vi "get folders.vi"(8 "error in":errorcluster, 11 "web service in":refnum<vi>) -> (0 "error out":errorcluster, 1 "web methods":refnum<vi>, 2 "startup":refnum<vi>, 3 "Web service project item out":refnum<vi>)   [LabVIEW 2013]
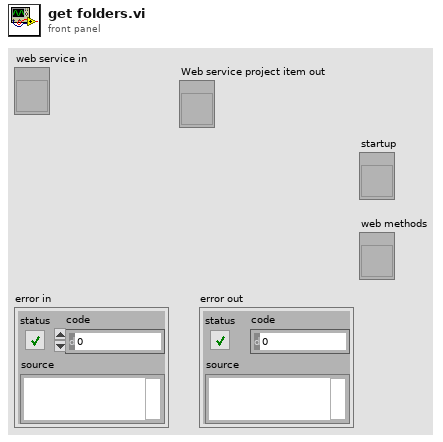
[diagram p1: front panel]
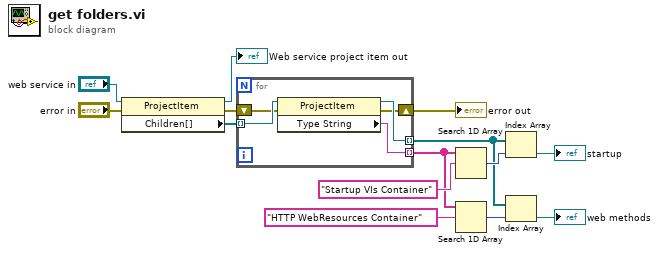
[diagram p0: block diagram]
diagram:
  n1 = property class="ProjectItem"(reference="web service in", error in="error in") -> (reference out=→"Web service project item out":refnum<vi>, error out=w12:errorcluster, "Children[]"=w13:refnum<vi>[])
  n2 = for {
    tunnel: w13 -> [w19] mode=indexing
    tunnel: [w18] -> w5 mode=indexing
    tunnel: [w17] -> w6 mode=indexing
    shift-right: [w16] -> w2
    shift-left: w12 -> [w15]
    n3 = property class="ProjectItem"(reference=w19, error in=w15) -> (reference out=w18:refnum<vi>, error out=w16:errorcluster, "Type String"=w17:string)
  }
  "error out" <- w2
  n4 = Search 1D Array(1D array=w6, element="Startup VIs Container" ("Type")) -> (index of element=w9:i32)  [unwired: 1 in]
  n5 = Search 1D Array(1D array=w6, element="HTTP WebResources Container" ("Type")) -> (index of element=w8:i32)  [unwired: 1 in]
  n6 = Index Array(array=w5, index=w9) -> (element=→"startup":refnum<vi>)
  n7 = Index Array(array=w5, index=w8) -> (element=→"web methods":refnum<vi>)
